vi "Parse Measurement.vi"(0 "Sample Field (on)":enum16{"off", "on"}(ring)=enum."on", 1 "Frequency Field (7)":i32=7 min=0 max=7, 2 "Capacitance Field (9)":i32=9 min=0 max=9, 3 "Loss Field (9)":i32=9 min=0 max=9, 5 "Voltage Field (on)":enum16{"off", "on"}(ring)=enum."on", 6 "Attentap Field (on)":enum16{"off", "on"}(ring)=enum."on", 7 "Error Messages (english)":enum16{"english", "numeric"}(ring), 8 "Measurement Line":string, 9 "Labeling (off)":enum16{"off", "on"}(ring)) -> (18 "Units":i32(ring) items=["", "nanosiemens", "dissipation factor", "kilohms", "gigohms", "loss vector (jpF)"], 19 "Error Code":i32, 20 "Sample":i32, 21 "Frequency":dbl, 22 "Capacitance":dbl format="%#_10f", 23 "Loss":dbl format="%#_10f", 24 "Loss Greater Than":bool, 25 "Voltage":dbl, 26 "Attentap":string, 27 "Error Message":string)   [LabVIEW 2019, in "Andeen-Hagerling 2700(400 firmware).lvlib"]
doc: "Parses a text line of measurement results from the bridge. Measurement results are dependent on the labelling parameter of Format and the Field parameters. Boolean inputs are provided to represent these parameters. These only need to be set if the the Format or Field are not set as in the Default Instrument Setup VI."
uses:
  Andeen-Hagerling 2700(400 firmware).lvlib
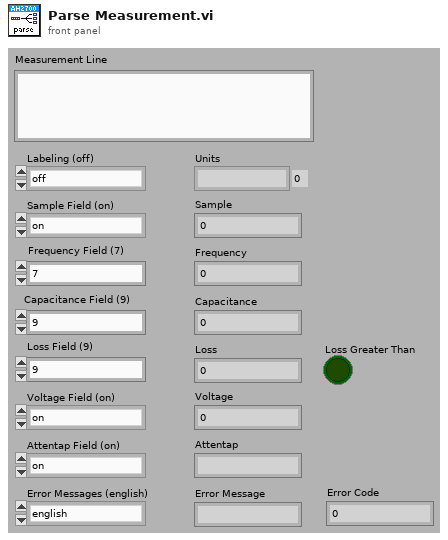
[diagram p1: front panel]
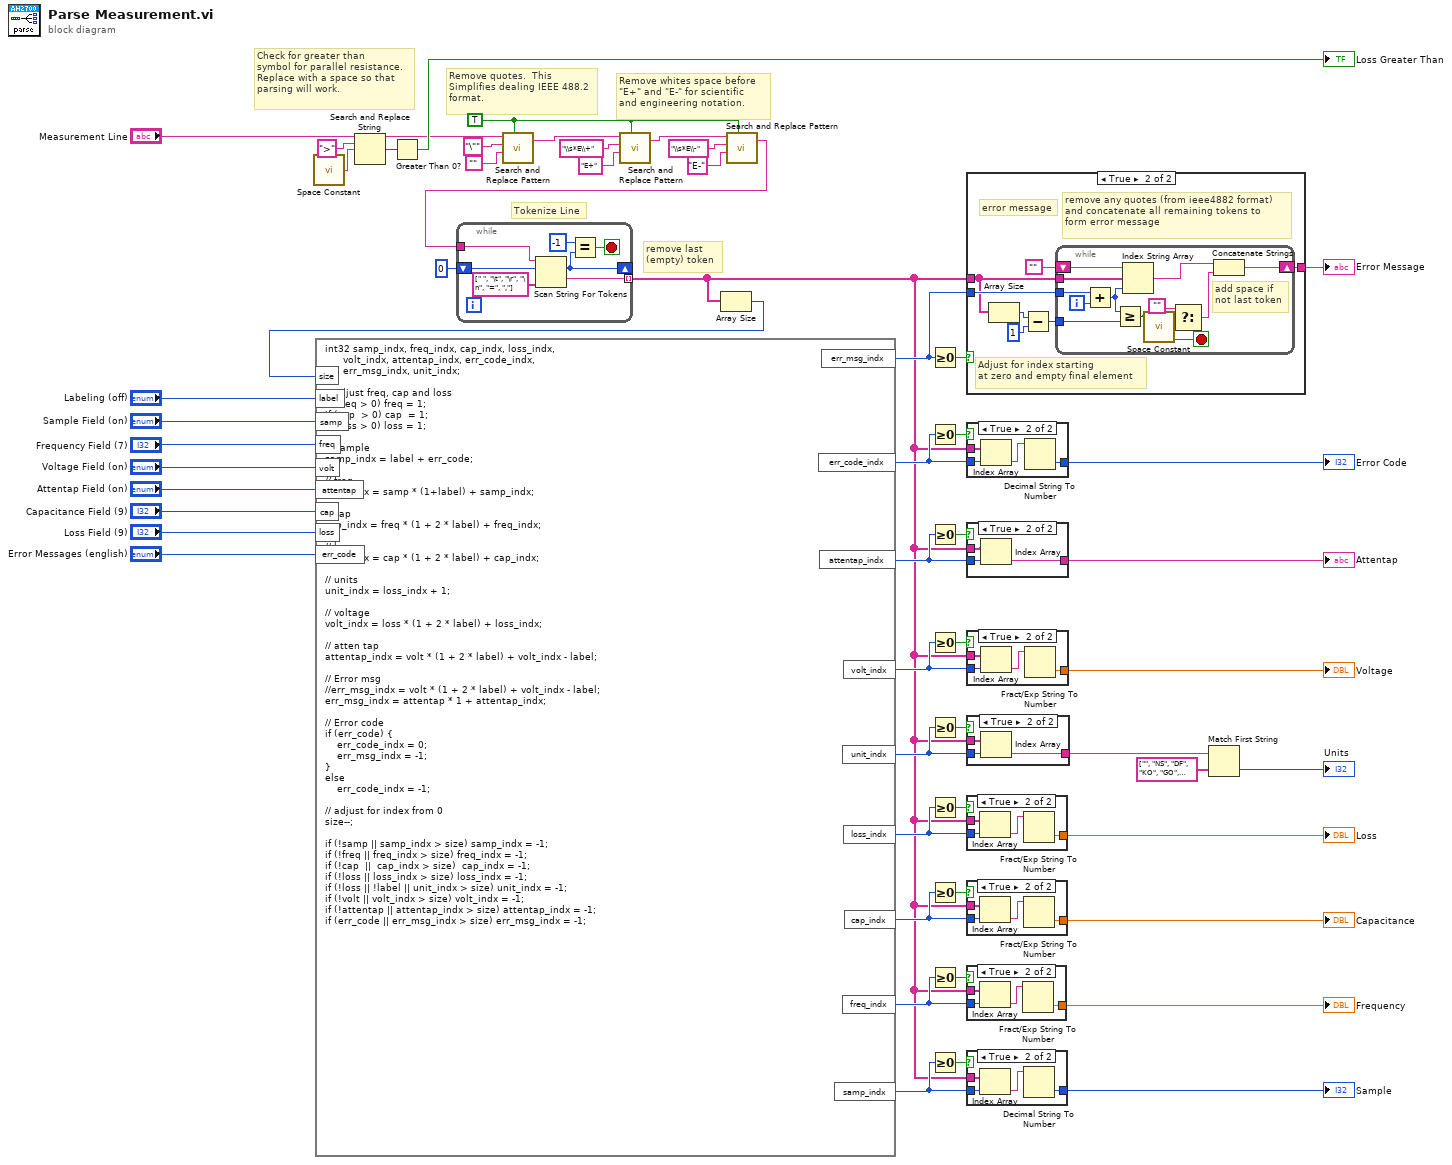
[diagram p0: block diagram]
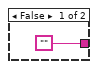
[diagram p2: hidden frame]
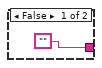
[diagram p3: hidden frame]
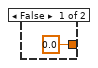
[diagram p4: hidden frame]
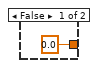
[diagram p5: hidden frame]
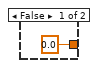
[diagram p6: hidden frame]
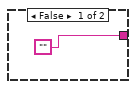
[diagram p7: hidden frame]
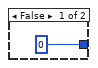
[diagram p8: hidden frame]
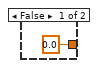
[diagram p9: hidden frame]
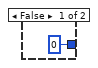
[diagram p10: hidden frame]
diagram:
  w15 = TRUE ("replace all? (F)")
  # "remove last\n(empty) token"
  # "Remove quotes.  This\nSimplifies dealing IEEE 488.2\nformat."
  # "Remove whites space before\n\"E+\" and \"E-\" for scientific\nand engineering notation."
  # "Tokenize Line"
  # "Check for greater than\nsymbol for parallel resistance.\nReplace with a space so that\nparsing will work."
  n1 = call <vilib>:"Space Constant.vi"() -> ("String"=w49:string)
  n2 = Search and Replace String(input string="Measurement Line", search string=">", replace string=w49) -> (result string=w14:string, number of replacements=w50:i32)  [unwired: 5 in, 2 out]
  n3 = Greater Than 0?(x=w50) -> (x > 0?=→"Loss Greater Than":bool)
  n4 = call <vilib>:"Search and Replace Pattern.vi"("string"=w14, "regular expression (\"\")"="\"" ("regular expression (\"\")"), "replace string (\"\")"="", "replace all? (F)"=w15) -> ("result string"=w18:string)  [unwired: 1 in, 1 out]
  n5 = call <vilib>:"Search and Replace Pattern.vi"("string"=w18, "regular expression (\"\")"="\\s*E\\+" ("regular expression (\"\")"), "replace string (\"\")"="E+" ("replace string (\"\")"), "replace all? (F)"=w15) -> ("result string"=w19:string)  [unwired: 1 in, 1 out]
  n6 = call <vilib>:"Search and Replace Pattern.vi"("string"=w19, "regular expression (\"\")"="\\s*E\\-" ("regular expression (\"\")"), "replace string (\"\")"="E-" ("replace string (\"\")"), "replace all? (F)"=w15) -> ("result string"=w13:string)  [unwired: 1 in, 1 out]
  n7 = while {
    tunnel: [w62] -> w1 mode=indexing
    tunnel: w13 -> [w61]
    shift-right: [w59] -> _
    shift-left: 0 ("token index") -> [w60]
    stop <- w63 stop-if-true
    n8 = Scan String For Tokens(6:string[] [" ", "\t", "\r", "\n", "=", ","] ("delimiters (\\s,\\t,\\r,\\n)"), 8:w60, 9:w61) -> (1:w62:string, 2:w59:i32)  [unwired: 3 in, 2 out]
    n9 = Equal?(x=-1 ("y"), y=w59) -> (x = y?=w63:bool)
  }
  n10 = Array Size(array=w1) -> (size(s)=w30:i32)
  n11 = formula code="int32 samp_indx, freq_indx, cap_indx, loss_indx, \n      volt_indx, attentap_indx, err_code_indx, \n      err_msg_indx, unit_indx;\n\n// adjust freq, cap and loss\nif (freq > 0) freq = 1;\nif (cap  > 0) cap  = 1;\nif (loss > 0) loss = 1;\n\n// Sample\nsamp_indx = label + err_code;\n\n// freq\nfreq_indx = samp * (1+label) + samp_indx;\n\n// cap\ncap_indx = freq * (1 + 2 * label) + freq_indx;\n\n// loss\nloss_indx = cap * (1 + 2 * label) + cap_indx;\n\n// units\nunit_indx = loss_indx + 1;\n\n// voltage\nvolt_indx = loss * (1 + 2 * label) + loss_indx;\n\n// atten tap\nattentap_indx = volt * (1 + 2 * label) + volt_indx - label;\n\n// Error msg\n//err_msg_indx = volt * (1 + 2 * label) + volt_indx - label;\nerr_msg_indx = attentap * 1 + attentap_indx;\n\n// Error code\nif (err_code) {\n    err_code_indx = 0;\n    err_msg_indx = -1;\n}\nelse\n    err_code_indx = -1;\n\n// adjust for index from 0\nsize--;\n\nif (!samp || samp_indx > size) samp_indx = -1;\nif (!freq || freq_indx > size) freq_indx = -1;\nif (!cap  ||  cap_indx > size)  cap_indx = -1;\nif (!loss || loss_indx > size) loss_indx = -1;\nif (!loss || !label || unit_indx > size) unit_indx = -1;\nif (!volt || volt_indx > size) volt_indx = -1;\nif (!attentap || attentap_indx > size) attentap_indx = -1;\nif (err_code || err_msg_indx > size) err_msg_indx = -1;"("samp"="Sample Field (on)", "label"="Labeling (off)", "err_code"="Error Messages (english)", "freq"="Frequency Field (7)", "cap"="Capacitance Field (9)", "loss"="Loss Field (9)", "volt"="Voltage Field (on)", "size"=w30, "attentap"="Attentap Field (on)") -> ("cap_indx"=w47:i32, "freq_indx"=w48:i32, "loss_indx"=w46:i32, "samp_indx"=w54:i32, "volt_indx"=w45:i32, "err_code_indx"=w53:i32, "err_msg_indx"=w52:i32, "unit_indx"=w44:i32, "attentap_indx"=w11:i32)
  n12 = Greater Or Equal To 0?(x=w52) -> (x >= 0?=w36:bool)
  n13 = Greater Or Equal To 0?(x=w53) -> (x >= 0?=w37:bool)
  n14 = Greater Or Equal To 0?(x=w11) -> (x >= 0?=w12:bool)
  n15 = Greater Or Equal To 0?(x=w45) -> (x >= 0?=w35:bool)
  n16 = Greater Or Equal To 0?(x=w44) -> (x >= 0?=w38:bool)
  n17 = Greater Or Equal To 0?(x=w46) -> (x >= 0?=w39:bool)
  n18 = Greater Or Equal To 0?(x=w47) -> (x >= 0?=w34:bool)
  n19 = Greater Or Equal To 0?(x=w48) -> (x >= 0?=w33:bool)
  n20 = Greater Or Equal To 0?(x=w54) -> (x >= 0?=w40:bool)
  n21 = case shown="True" w36 {
    tunnel: w1 -> [_ w70]
    tunnel: w52 -> [_ w71]
    tunnel: ["" w69] -> w56
    frame False {
    }
    frame True {
      # "Adjust for index starting\nat zero and empty final element"
      # "error message"
      # "remove any quotes (from ieee4882 format)\nand concatenate all remaining tokens to \nform error message"
      n22 = Array Size(array=w70) -> (size(s)=w67:i32)
      n23 = Subtract(x=w67, y=1) -> (x-y=w68:i32)
      n24 = while {
        tunnel: w71 -> [w82]
        tunnel: w70 -> [w83]
        tunnel: w68 -> [w79]
        shift-right: [w78] -> w69
        shift-left: "" -> [w73]
        i -> [w81]
        stop <- w74 stop-if-true
        # "add space if\nnot last token"
        n25 = Add(x=w82, y=w81) -> (x+y=w80:i32)
        n26 = Greater Or Equal?(x=w80, y=w79) -> (x >= y?=w74:bool)
        n27 = Index String Array(1:w80, 2:w83, 3:w73) -> (0:w72:string)
        n28 = call <vilib>:"Space Constant.vi"() -> ("String"=w75:string)
        n29 = Select(t="", s=w74, f=w75) -> (s? t:f=w76:string)
        n30 = Concatenate Strings(w72, w76) -> (w78:string)
      }
    }
  }
  "Error Message" <- w56
  n31 = case shown="True" w37 {
    tunnel: w1 -> [_ w88]
    tunnel: w53 -> [_ w86]
    tunnel: [0 w85] -> w55
    frame False {
    }
    frame True {
      n32 = Index Array(array=w88, index=w86) -> (element=w87:string)
      n33 = Decimal String To Number(string=w87) -> (number=w85:i32)  [unwired: 2 in, 1 out]
    }
  }
  "Error Code" <- w55
  n34 = case shown="True" w12 {
    tunnel: w1 -> [_ w92]
    tunnel: w11 -> [_ w91]
    tunnel: ["" w90] -> w10
    frame False {
    }
    frame True {
      n35 = Index Array(array=w92, index=w91) -> (element=w90:string)
    }
  }
  "Attentap" <- w10
  n36 = case shown="True" w35 {
    tunnel: w1 -> [_ w96]
    tunnel: w45 -> [_ w95]
    tunnel: [0.0 w97] -> w28
    frame False {
    }
    frame True {
      n37 = Index Array(array=w96, index=w95) -> (element=w94:string)
      n38 = Fract/Exp String To Number(string=w94) -> (number=w97:dbl)  [unwired: 3 in, 1 out]
    }
  }
  "Voltage" <- w28
  n39 = case shown="True" w38 {
    tunnel: w1 -> [_ w101]
    tunnel: w44 -> [_ w100]
    tunnel: ["" w99] -> w27
    frame False {
    }
    frame True {
      n40 = Index Array(array=w101, index=w100) -> (element=w99:string)
    }
  }
  n41 = case shown="True" w39 {
    tunnel: w1 -> [_ w105]
    tunnel: w46 -> [_ w104]
    tunnel: [0.0 w106] -> w41
    frame False {
    }
    frame True {
      n42 = Index Array(array=w105, index=w104) -> (element=w103:string)
      n43 = Fract/Exp String To Number(string=w103) -> (number=w106:dbl)  [unwired: 3 in, 1 out]
    }
  }
  "Loss" <- w41
  n44 = case shown="True" w34 {
    tunnel: w1 -> [_ w110]
    tunnel: w47 -> [_ w109]
    tunnel: [0.0 w111] -> w42
    frame False {
    }
    frame True {
      n45 = Index Array(array=w110, index=w109) -> (element=w108:string)
      n46 = Fract/Exp String To Number(string=w108) -> (number=w111:dbl)  [unwired: 3 in, 1 out]
    }
  }
  "Capacitance" <- w42
  n47 = case shown="True" w33 {
    tunnel: w1 -> [_ w115]
    tunnel: w48 -> [_ w114]
    tunnel: [0.0 w116] -> w32
    frame False {
    }
    frame True {
      n48 = Index Array(array=w115, index=w114) -> (element=w113:string)
      n49 = Fract/Exp String To Number(string=w113) -> (number=w116:dbl)  [unwired: 3 in, 1 out]
    }
  }
  "Frequency" <- w32
  n50 = case shown="True" w40 {
    tunnel: w1 -> [_ w121]
    tunnel: w54 -> [_ w120]
    tunnel: [0 w118] -> w43
    frame False {
    }
    frame True {
      n51 = Index Array(array=w121, index=w120) -> (element=w119:string)
      n52 = Decimal String To Number(string=w119) -> (number=w118:i32)  [unwired: 2 in, 1 out]
    }
  }
  "Sample" <- w43
  n53 = Match First String(2:string[] ["", "NS", "DF", "KO", "GO", "JP"] ("string array"), 3:w27) -> (0:→"Units":i32)  [unwired: 1 out]
